vi "FTT_V2.1_dll.vi"(0 "data":dbl[][](array[numeric]), 1 "index":dbl[](array[numeric]), 2 "power":dbl=0.01 min=0.01 max=1.0 step=0.01, 3 "alpha":dbl min=0.0 max=1.0 step=0.01, 5 "input cluster":T1, 7 "Blur_int":i32=1, 9 "buffer in":dbl[][](array[numeric]), 11 "error in (no error)":errorcluster, 12 "interp_value":i32=5, 14 "# of Cores":i32=1) -> (4 "Depth_profile":dbl[][](array[numeric]), 6 "complex_depth_profile":dbl[][](array[numeric]), 10 "buffer out":dbl[][](array[numeric]), 15 "error out":errorcluster)   [LabVIEW 2019]
uses:
  SD_OCT_DLL_Ver2.1.dll
panel:
  in  "Blur_coef":dbl=2.0
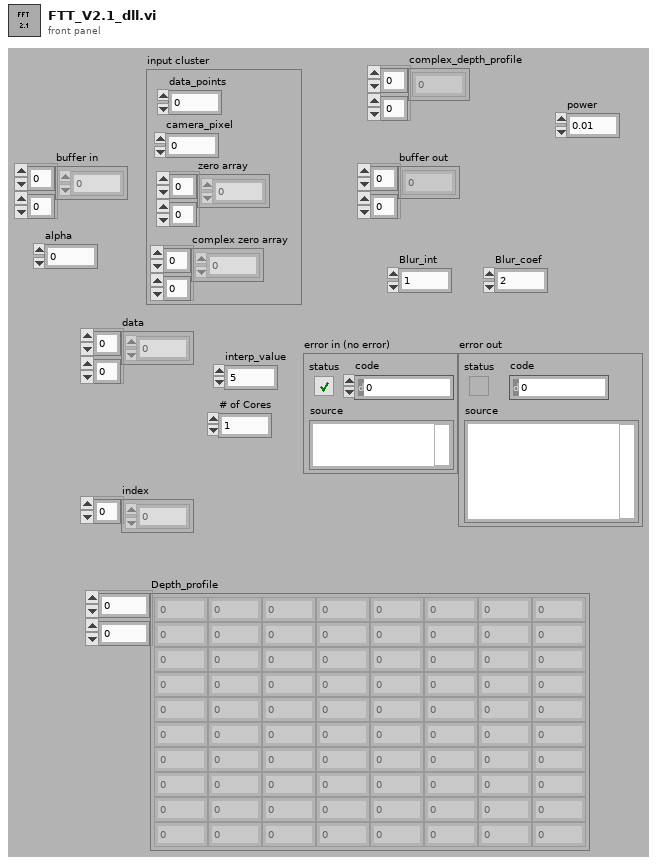
[diagram p1: front panel]
types:
  T1 = cluster{"data_points":i32, "camera_pixel":i32, "zero array":dbl[][], "complex zero array":dbl[][]}
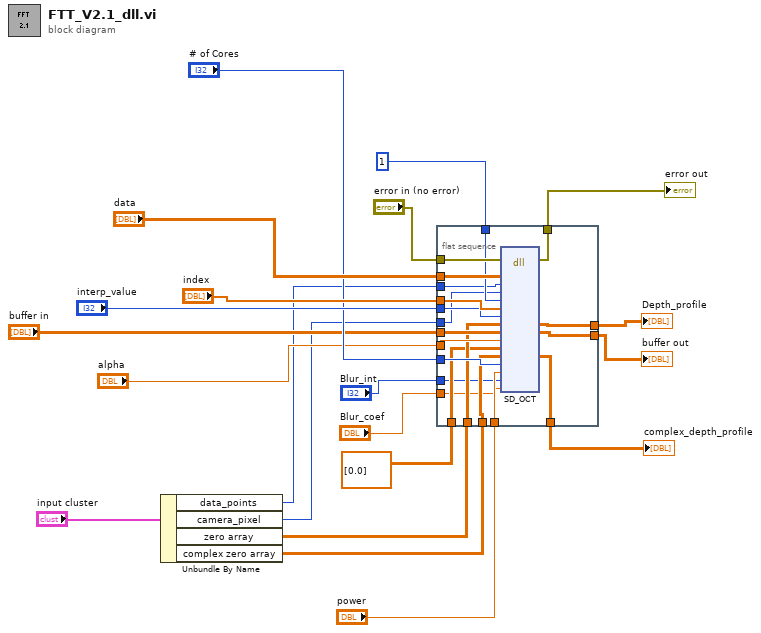
[diagram p0: block diagram]
diagram:
  n1 = Unbundle By Name("input cluster") -> ("data_points"=w8:i32, "camera_pixel"=w7:i32, "zero array"=w6:dbl[][], "complex zero array"=w5:dbl[][])
  n2 = flat-sequence {
    tunnel: "data" -> [w41]
    tunnel: "index" -> [w40]
    tunnel: [w39] -> w19
    tunnel: [w38] -> w18
    tunnel: "interp_value" -> [w37]
    tunnel: "error in (no error)" -> [w36]
    tunnel: "# of Cores" -> [w35]
    tunnel: 1 ("Magnification") -> [w34]
    tunnel: [w33] -> w13
    tunnel: "buffer in" -> [w32]
    tunnel: "alpha" -> [w31]
    tunnel: [w30] -> w10
    tunnel: w8 -> [w29]
    tunnel: w7 -> [w28]
    tunnel: w6 -> [w27]
    tunnel: w5 -> [w26]
    tunnel: dbl[][] [[0.0]] ("complex zero array") -> [w25]
    tunnel: "power" -> [w24]
    tunnel: "Blur_int" -> [w23]
    tunnel: "Blur_coef" -> [w22]
    frame #0 {
      n3 = dll-call lib="C:/Users/hesfandi/Desktop/labview/LabViewCode/SD_OCT_DLL_Ver2.1.dll" fn="SD_OCT"(error in=w36, "Data"=w41, "data_points"=w29, "camera_pixel"=w28, "Magnification"=w34, "new_index"=w40, "interp_value"=w37, "depth_profile"=w27, "buffer"=w32, "alpha"=w31, "weight"=w25, "complex_depth_profile"=w26, "core_number"=w35, "power"=w24, "Blur_int"=w23, "Blur_coef"=w22) -> (error out=w39:errorcluster, "depth_profile"=w38:dbl[][], "buffer"=w33:dbl[][], "complex_depth_profile"=w30:dbl[][])  [unwired: 15 in, 1 out]
    }
  }
  "error out" <- w19
  "Depth_profile" <- w18
  "buffer out" <- w13
  "complex_depth_profile" <- w10
